vi "Get Orientation.vi"(0 "Matches (pixel)":T2(array[cluster]) {"Bounding Box"."y" format="%.2f"; "Bounding Box"."x" format="%.2f"; "Position"."y" format="%.2f"; "Position"."x" format="%.2f"; "Score" format="%.2f"; "Scale" format="%.2f"; "Angle" format="%.2f"}, 2 "Image Src":T1, 5 "error in (no error)":errorcluster, 6 "Image Dst":T1(plugin-control), 7 "y":dbl=20.0 format="%#_13g", 9 "X":dbl=100.0 format="%#_13g", 11 "yB":dbl=20.0, 13 "XB":dbl=100.0 format="%#_13g") -> (10 "Centre":dbl[][](array[numeric]) format="%.2f", 12 "Angle":sgl, 14 "Image 3":T1(plugin-control), 15 "X":sgl, 16 "no error":bool, 18 "y":sgl, 19 "错误输出":errorcluster)   [LabVIEW 2016]
uses:
  <vilib>/vision/Image Controls.llb/IMAQ Image.ctl
  <vilib>/vision/Measure.llb/Edge Options.ctl
  <vilib>/vision/Measure.llb/Edge Polarity.ctl
  <vilib>/vision/Measure.llb/Straight Edge Options.ctl
  <vilib>/vision/Measure.llb/Straight Edge Process.ctl
  <vilib>/vision/NI_Vision_Development_Module.lvlib
panel:
  out "Image 2":T1(plugin-control)
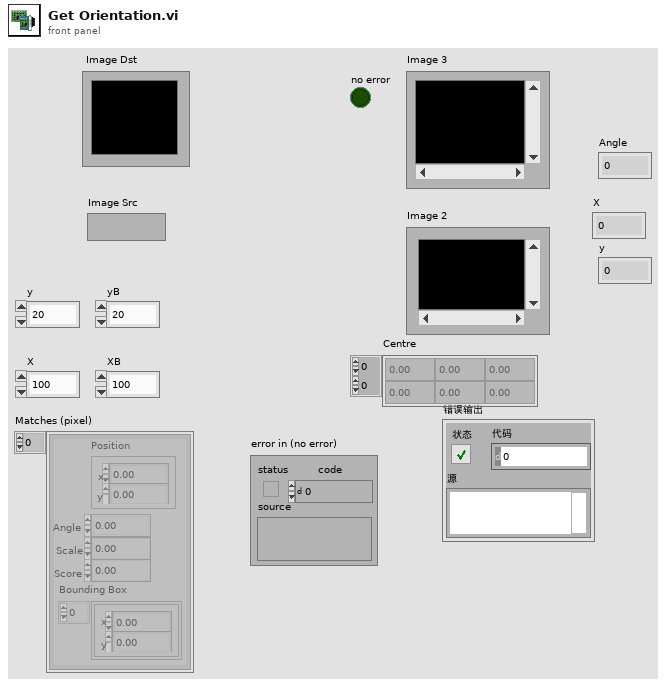
[diagram p1: front panel]
types:
  T1 = typedef "IMAQ Image.ctl" = refnum<image>
  T2 = cluster{"Position":cluster{"x":sgl, "y":sgl}, "Angle":sgl, "Scale":sgl, "Score":sgl, "Bounding Box":cluster{"x":sgl, "y":sgl}[]}[]
  T3 = cluster{"Feature":u32, "Points IDs":cluster{"GUID":string, "Index":i32}[]}[]
  T4 = typedef "IMAQ Rectangle" = cluster{"Left":i32, "Top":i32, "Right":i32, "Bottom":i32, "Rotation":dbl}
  T5 = typedef "Straight Edge Options.ctl" = cluster{"Number of Lines":i32, "Type":T6, "Min. Score":dbl, "Max. Score":dbl, "Orientation":dbl, "Angle Range":dbl, "Angle Tolerance":dbl, "Step Size":u32, "Min. SNR (db)":dbl, "Min. Points (%)":dbl, "Hough Iterations":i32}
  T6 = typedef "Straight Edge Process.ctl" = enum32{"First Edge Rake", "Best Edge Rake", "Hough Edge Rake", "First Edge Projection", "Best Edge Projection"}
  T7 = typedef "Edge Options.ctl" = cluster{"Edge Polarity":T8, "Kernel Size":u32, "Width":u32, "Minimum Edge Strength":sgl, "Interpolation Type":enum32{"Zero Order", "Bilinear", "Quadratic", "Cubic", "Bilinear Fixed"}, "Data Processing Method":enum32{"Average", "Median"}}
  T8 = typedef "Edge Polarity.ctl" = u32
  T9 = cluster{"Search Direction":u32, "Edge Options":T7, "Show Search Area":bool, "Show Search Lines":bool, "Show Edges Found":bool, "Show Result":bool, "Search Area Color":u32, "Search Lines Color":u32, "Edge Locations Color":u32, "Result Color":u32, "Overlay Group Name":string}
  T10 = typedef "Particle Parameters" = i32
  T11 = cluster{"Measurement Parameter":T10, "Range Lower Value":dbl, "Range Upper Value":dbl, "Range":bool, "Measurement Type":bool}[]
  T12 = cluster{"Position":cluster{"x":sgl, "y":sgl}, "Angle":sgl, "Scale":sgl, "Score":sgl, "Bounding Box":cluster{"x":sgl, "y":sgl}[]}
  T13 = typedef "ROI Descriptor" = cluster{"Global Rectangle":i32[], "Contours":cluster{"ID":enum32{"External", "Internal"}, "Type":u32, "Coordinates":i32[]}[]}
  T14 = cluster{"histogram":u32[], "Minimal Value":sgl, "Maximal Value":sgl, "Starting Value":sgl, "Interval Width":sgl, "Mean Value":sgl, "Standard  Variation":sgl, "Area (pixels)":i32}
  T15 = typedef "Image Type" = u32
  T16 = cluster{"Point1 (Pixels)":cluster{"X":sgl, "Y":sgl}, "Point2 (Pixels)":cluster{"X":sgl, "Y":sgl}, "Point1 (Real-World)":cluster{"X":sgl, "Y":sgl}, "Point2 (Real-World)":cluster{"X":sgl, "Y":sgl}, "Angle (Pixel)":dbl, "Angle (Real-World)":dbl, "Score":dbl, "Straightness":dbl, "Average SNR (db)":dbl, "Calibration Valid":bool}[]
  T17 = cluster{"Point1 (Pixels)":cluster{"X":sgl, "Y":sgl}, "Point2 (Pixels)":cluster{"X":sgl, "Y":sgl}, "Point1 (Real-World)":cluster{"X":sgl, "Y":sgl}, "Point2 (Real-World)":cluster{"X":sgl, "Y":sgl}, "Angle (Pixel)":dbl, "Angle (Real-World)":dbl, "Score":dbl, "Straightness":dbl, "Average SNR (db)":dbl, "Calibration Valid":bool}
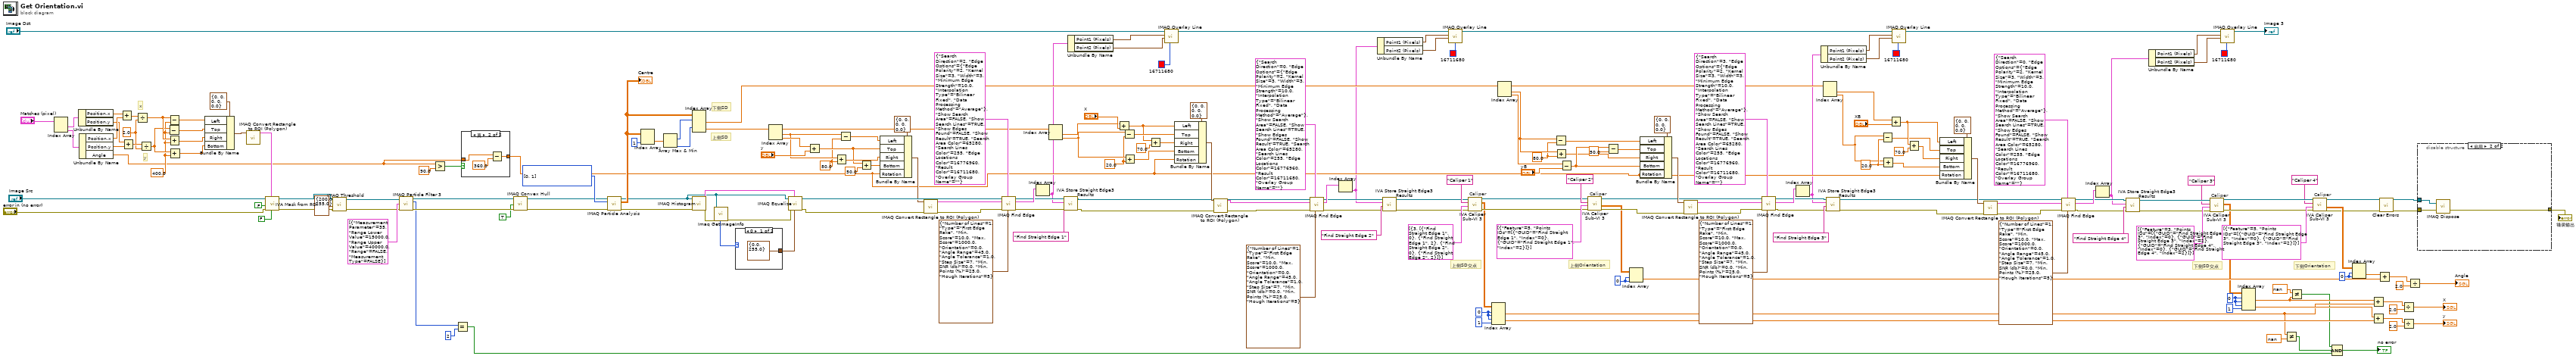
[diagram p0: block diagram]
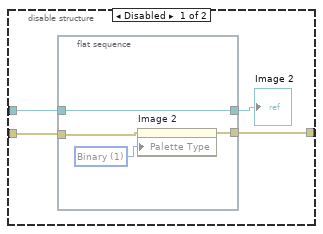
[diagram p2: hidden frame]
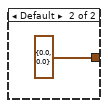
[diagram p4: hidden frame]
diagram:
  w52 = 0 ("索引 (行)")
  w50 = 0 ("索引 (行)")
  w59 = 0
  w60 = 0
  w79 = 20.0 ("y")
  w104 = 80.0 ("y")
  w106 = 20.0 ("y")
  w107 = 80.0 ("y")
  w185 = T10[] [0, 1] items=["Center of Mass X", "Center of Mass Y", "First Pixel X", "First Pixel Y", "Bounding Rect Left", "Bounding Rect Top", "Bounding Rect Right", "Bounding Rect Bottom", "Max Feret Diameter Start X", "Max Feret Diameter Start Y", "Max Feret Diameter End X", "Max Feret Diameter End Y", "Max Horiz. Segment Length Left", "Max Horiz. Segment Length Right", "Max Horiz. Segment Length Row", "-", "Bounding Rect Width", "Bounding Rect Height", "Bounding Rect Diagonal", "Perimeter", "Convex Hull Perimeter", "Holes' Perimeter", "Max Feret Diameter", "Equivalent Ellipse Major Axis", "Equivalent Ellipse Minor Axis", "Equivalent Ellipse Minor Axis (Feret)", "Equivalent Rect Long Side", "Equivalent Rect Short Side", "Equivalent Rect Diagonal", "Equivalent Rect Short Side (Feret)", "Average Horiz. Segment Length", "Average Vert. Segment Length", "Hydraulic Radius", "Waddel Disk Diameter", "-", "Area", "Holes' Area", "Particle & Holes' Area", "Convex Hull Area", "Image Area", "-", "Number of Holes", "Number of Horiz. Segments", "Number of Vert. Segments", "-", "Orientation", "Max Feret Diameter Orientation", "-", "% Area/Image Area", "% Area/(Particle & Holes' Area)", "Ratio of Equivalent Ellipse Axes", "Ratio of Equivalent Rect Sides", "-", "Elongation Factor", "Compactness Factor", "Heywood Circularity Factor", "Type Factor", "-", "Sum X", "Sum Y", "Sum XX", "Sum XY", "Sum YY", "Sum XXX", "Sum XXY", "Sum XYY", "Sum YYY", "-", "Moment of Inertia XX", "Moment of Inertia XY", "Moment of Inertia YY", "Moment of Inertia XXX", "Moment of Inertia XXY", "Moment of Inertia XYY", "Moment of Inertia YYY", "Norm. Moment of Inertia XX", "Norm. Moment of Inertia XY", "Norm. Moment of Inertia YY", "Norm. Moment of Inertia XXX", "Norm. Moment of Inertia XXY", "Norm. Moment of Inertia XYY", "Norm. Moment of Inertia YYY", "Hu Moment 1", "Hu Moment 2", "Hu Moment 3", "Hu Moment 4", "Hu Moment 5", "Hu Moment 6", "Hu Moment 7"] ("Pixel Measurements")
  w197 = sgl 400.0 ("y")
  w204 = sgl 2.0 ("y")
  # "下侧Orientation"
  # "下侧SD交点"
  # "Caliper"
  # "Caliper"
  # "上侧Orientation"
  # "上侧SD交点"
  # "Caliper"
  # "Caliper"
  # "下侧SD"
  # "上侧SD"
  # "y"
  # "x"
  n1 = Index Array(array="Matches (pixel)") -> (element #1=w212:T12, element #2=w211:T12)  [unwired: 2 in]
  n2 = Unbundle By Name(w212) -> ("Position.x"=w209:sgl, "Position.y"=w208:sgl)
  n3 = Unbundle By Name(w211) -> ("Position.x"=w210:sgl, "Position.y"=w207:sgl, "Angle"=w154:sgl)
  n4 = Add(x=w209, y=w210) -> (x+y=w206:sgl)
  n5 = Add(x=w208, y=w207) -> (x+y=w205:sgl)
  n6 = Divide(x=w206, y=w204) -> (x/y=w199:sgl)
  n7 = Divide(x=w205, y=w204) -> (x/y=w198:sgl)
  n8 = Subtract(x=w198, y=w197) -> (x-y=w200:sgl)
  n9 = Subtract(x=w199, y=w197) -> (x-y=w201:sgl)
  n10 = Add(x=w199, y=w197) -> (x+y=w196:sgl)
  n11 = Add(x=w198, y=w197) -> (x+y=w195:sgl)
  n12 = Bundle By Name(cluster=T4 {"Left"=0, "Top"=0, "Right"=0, "Bottom"=0, "Rotation"=0.0} ("Rectangle"), "Left"=w201, "Top"=w200, "Right"=w196, "Bottom"=w195) -> (w202:T4)
  n13 = call "IMAQ Convert Rectangle to ROI (Polygon)"("Rectangle"=w202) -> ("ROI Descriptor"=w194:T13)  [unwired: 7 in, 2 out]
  n14 = call <vilib>:"IVA Mask from ROI.vi"("Shrink"=FALSE ("Out / In"), "ROI Descriptor"=w194, "error in (no error)"="error in (no error)", "Out / In"=FALSE, "Image Src"="Image Src") -> ("error out"=w16:errorcluster, "Image Out"=w14:T1)  [unwired: 5 out]
  n15 = call "IMAQ Threshold"("error in (no error)"=w16, "Range"=cluster{"Lower value":sgl, "Upper value":sgl} {"Lower value"=200.0, "Upper value"=255.0}, "Image Src"=w14) -> ("error out"=w17:errorcluster, "Image Dst Out"=w15:T1)  [unwired: 7 in]
  n16 = call "IMAQ Particle Filter 3"("Image Src"=w15, "Selection Values"=T11 [{"Measurement Parameter"=35, "Range Lower Value"=15000.0, "Range Upper Value"=40000.0, "Range"=FALSE, "Measurement Type"=FALSE}], "error in (no error)"=w17) -> ("Image Dst Out"=w188:T1, "Number of Particles"=w13:i32, "error out"=w187:errorcluster)  [unwired: 10 in]
  n17 = Greater?(x=w154, y=sgl 90.0) -> (0:w155:bool)
  n18 = Equal?(x=w13, y=2) -> (x = y?=w1:bool)
  n19 = case shown="真" w155 {
    tunnel: w154 -> [w213 w214]
    tunnel: [w213 w216] -> w74
    frame False {
    }
    frame True {
      n20 = Subtract(x=w214, y=360.0 ("x")) -> (x-y=w216:dbl)
    }
  }
  n21 = call "IMAQ Convex Hull"("error in (no error)"=w187, "Connectivity 4/8 (8)"=TRUE, "Image Src"=w188) -> ("error out"=w183:errorcluster, "Image Dst Out"=w184:T1)  [unwired: 7 in]
  n22 = call "IMAQ Particle Analysis"("error in (no error)"=w183, "Pixel Measurements"=w185, "Image"=w184) -> ("error out"=w172:errorcluster, "Particle Measurements (Pixels)"=w180:dbl[][], "Image Out (duplicate)"=w171:T1)  [unwired: 3 in, 3 out]
  "Centre" <- w180
  n23 = Index Array(array=w180, index (col)=1 ("禁用的索引 (列)")) -> (element=w181:dbl[])  [unwired: 1 in]
  n24 = Array Max & Min(array=w181) -> (max index (indices)=w179:i32, min index (indices)=w178:i32)  [unwired: 2 out]
  n25 = Index Array(array=w180, index (row) #1=w179, index (row) #2=w178) -> (element #1=w82:dbl[], element #2=w144:dbl[])  [unwired: 2 in]
  n26 = call "IMAQ Histogram"("error in (no error)"=w172, "Image"=w171) -> ("error out"=w175:errorcluster, "Histogram Report"=w177:T14)  [unwired: 3 in, 5 out]
  n27 = call "Imaq GetImageInfo"("error in (no error)"=w175, "Image"=w171) -> ("error out"=w174:errorcluster, "Image Type"=w176:T15)  [unwired: 8 out]
  n28 = case "条件结构" shown="0" w176 {
    tunnel: [cluster{"Minimum":sgl, "Maximum":sgl} {"Minimum"=0.0, "Maximum"=255.0} ("Range") cluster{"Minimum":sgl, "Maximum":sgl} {"Minimum"=0.0, "Maximum"=0.0} ("Range")] -> w173
    frame 0 {
    }
    frame Default {
    }
  }
  n29 = Index Array(array=w144) -> (element #1=w161:dbl, element #2=w162:dbl)  [unwired: 2 in]
  n30 = call "IMAQ Equalize"("Range"=w173, "Histogram Report"=w177, "error in (no error)"=w174, "Image Src"=w171) -> ("error out"=w167:errorcluster, "Image Dst Out"=w170:T1)  [unwired: 2 in, 4 out]
  n31 = Add(x=w162, y="y") -> (x+y=w158:dbl)
  n32 = Add(x=w161, y=w107) -> (x+y=w160:dbl)
  n33 = Subtract(x=w161, y=w107) -> (x-y=w164:dbl)
  n34 = Add(x=w158, y=50.0) -> (x+y=w157:dbl)
  n35 = Bundle By Name(cluster=T4 {"Left"=0, "Top"=0, "Right"=0, "Bottom"=0, "Rotation"=0.0} ("Rectangle"), "Left"=w164, "Top"=w158, "Right"=w160, "Bottom"=w157, "Rotation"=w74) -> (w165:T4)
  n36 = call "IMAQ Convert Rectangle to ROI (Polygon)"("error in (no error)"=w167, "Rectangle"=w165) -> ("error out"=w152:errorcluster, "ROI Descriptor"=w153:T13)  [unwired: 6 in, 1 out]
  n37 = call "IMAQ Find Edge"("Line Fit Options"=T5 {"Number of Lines"=1, "Type"=enum."First Edge Rake", "Min. Score"=10.0, "Max. Score"=1000.0, "Orientation"=0.0, "Angle Range"=45.0, "Angle Tolerance"=1.0, "Step Size"=7, "Min. SNR (db)"=0.0, "Min. Points (%)"=25.0, "Hough Iterations"=5}, "Options"=T9 {"Search Direction"=2, "Edge Options"={"Edge Polarity"=2, "Kernel Size"=3, "Width"=3, "Minimum Edge Strength"=10.0, "Interpolation Type"=enum."Bilinear Fixed", "Data Processing Method"=enum."Average"}, "Show Search Area"=FALSE, "Show Search Lines"=TRUE, "Show Edges Found"=FALSE, "Show Result"=TRUE, "Search Area Color"=65280, "Search Lines Color"=255, "Edge Locations Color"=16776960, "Result Color"=16711680, "Overlay Group Name"=""}, "error in (no error)"=w152, "ROI Descriptor"=w153, "Image"=w170) -> ("error out"=w148:errorcluster, "Straight Edges"=w151:T16, "Image Out"=w150:T1)  [unwired: 1 in, 3 out]
  n38 = Index Array(array=w151) -> (element=w40:T17)  [unwired: 1 in]
  n39 = Index Array(array=w144) -> (element #1=w140:dbl, element #2=w143:dbl)  [unwired: 2 in]
  n40 = call <vilib>:"IVA Store Straight Edge3 Results.vi"("error in (no error)"=w148, "Step Name"="Find Straight Edge 1", "Straight Edge"=w40, "Image in"=w150) -> ("error out"=w147:errorcluster, "Image dup"=w135:T1)  [unwired: 1 in, 5 out]
  n41 = Unbundle By Name(w40) -> ("Point1 (Pixels)"=w39:cluster{"X":sgl, "Y":sgl}, "Point2 (Pixels)"=w38:cluster{"X":sgl, "Y":sgl})
  n42 = Add(x=w140, y="X") -> (x+y=w123:dbl)
  n43 = Subtract(x=w143, y=w106) -> (x-y=w124:dbl)
  n44 = Add(x=w143, y=w106) -> (x+y=w138:dbl)
  n45 = Add(x=w123, y=70.0) -> (x+y=w139:dbl)
  n46 = call "IMAQ Overlay Line"("Color"=u32 16711680, "End Point"=w38, "Start Point"=w39, "Image"="Image Dst") -> ("Image Out"=w32:T1)  [unwired: 6 in, 1 out]
  n47 = Bundle By Name(cluster=T4 {"Left"=0, "Top"=0, "Right"=0, "Bottom"=0, "Rotation"=0.0} ("Rectangle"), "Left"=w123, "Top"=w124, "Right"=w139, "Bottom"=w138, "Rotation"=w74) -> (w145:T4)
  n48 = call "IMAQ Convert Rectangle to ROI (Polygon)"("error in (no error)"=w147, "Rectangle"=w145) -> ("error out"=w136:errorcluster, "ROI Descriptor"=w137:T13)  [unwired: 6 in, 1 out]
  n49 = call "IMAQ Find Edge"("Line Fit Options"=T5 {"Number of Lines"=1, "Type"=enum."First Edge Rake", "Min. Score"=10.0, "Max. Score"=1000.0, "Orientation"=0.0, "Angle Range"=45.0, "Angle Tolerance"=1.0, "Step Size"=7, "Min. SNR (db)"=0.0, "Min. Points (%)"=25.0, "Hough Iterations"=5}, "Options"=T9 {"Search Direction"=0, "Edge Options"={"Edge Polarity"=2, "Kernel Size"=3, "Width"=3, "Minimum Edge Strength"=10.0, "Interpolation Type"=enum."Bilinear Fixed", "Data Processing Method"=enum."Average"}, "Show Search Area"=FALSE, "Show Search Lines"=TRUE, "Show Edges Found"=FALSE, "Show Result"=TRUE, "Search Area Color"=65280, "Search Lines Color"=255, "Edge Locations Color"=16776960, "Result Color"=16711680, "Overlay Group Name"=""}, "error in (no error)"=w136, "ROI Descriptor"=w137, "Image"=w135) -> ("error out"=w126:errorcluster, "Straight Edges"=w132:T16, "Image Out"=w131:T1)  [unwired: 1 in, 3 out]
  n50 = Index Array(array=w132) -> (element=w35:T17)  [unwired: 1 in]
  n51 = Unbundle By Name(w35) -> ("Point1 (Pixels)"=w34:cluster{"X":sgl, "Y":sgl}, "Point2 (Pixels)"=w33:cluster{"X":sgl, "Y":sgl})
  n52 = call <vilib>:"IVA Store Straight Edge3 Results.vi"("error in (no error)"=w126, "Step Name"="Find Straight Edge 2", "Straight Edge"=w35, "Image in"=w131) -> ("error out"=w125:errorcluster, "Image dup"=w127:T1)  [unwired: 1 in, 5 out]
  n53 = call "IMAQ Overlay Line"("Color"=u32 16711680, "End Point"=w33, "Start Point"=w34, "Image"=w32) -> ("Image Out"=w27:T1)  [unwired: 6 in, 1 out]
  n54 = call <vilib>:"IVA Caliper Sub-VI 3.vi"("error in"=w125, "Parameters"=T3 [{"Feature"=3, "Points IDs"=[{"GUID"="Find Straight Edge 1", "Index"=0}, {"GUID"="Find Straight Edge 1", "Index"=2}, {"GUID"="Find Straight Edge 2", "Index"=0}, {"GUID"="Find Straight Edge 2", "Index"=2}]}], "Step Name"="Caliper 1", "Image In"=w127) -> ("error out"=w119:errorcluster, "Results (Pixels)"=w53:sgl[][], "Image Out"=w118:T1)  [unwired: 1 in, 4 out]
  n55 = Index Array(array=w53, index (row) #1=w52, index (col) #1=w52, index (row) #2=w52, index (col) #2=1 ("索引 (行)")) -> (element #1=w5:sgl, element #2=w43:sgl)
  n56 = Index Array(array=w82) -> (element #1=w105:dbl, element #2=w101:dbl)  [unwired: 2 in]
  n57 = Subtract(x=w105, y=w104) -> (x-y=w97:dbl)
  n58 = Add(x=w105, y=w104) -> (x+y=w96:dbl)
  n59 = Subtract(x=w101, y="yB") -> (x-y=w99:dbl)
  n60 = call <vilib>:"IVA Caliper Sub-VI 3.vi"("error in"=w119, "Parameters"=T3 [{"Feature"=5, "Points IDs"=[{"GUID"="Find Straight Edge 1", "Index"=0}, {"GUID"="Find Straight Edge 1", "Index"=2}]}], "Step Name"="Caliper 2", "Image In"=w118) -> ("error out"=w102:errorcluster, "Results (Calibrated)"=w61:sgl[][], "Image Out"=w103:T1)  [unwired: 1 in, 4 out]
  n61 = Subtract(x=w99, y=50.0) -> (x-y=w98:dbl)
  n62 = Index Array(array=w61, index (row)=w60, index (col)=w60) -> (element=w57:sgl)
  n63 = Bundle By Name(cluster=T4 {"Left"=0, "Top"=0, "Right"=0, "Bottom"=0, "Rotation"=0.0} ("Rectangle"), "Left"=w97, "Top"=w98, "Right"=w96, "Bottom"=w99, "Rotation"=w74) -> (w114:T4)
  n64 = call "IMAQ Convert Rectangle to ROI (Polygon)"("error in (no error)"=w102, "Rectangle"=w114) -> ("error out"=w112:errorcluster, "ROI Descriptor"=w113:T13)  [unwired: 6 in, 1 out]
  n65 = call "IMAQ Find Edge"("Line Fit Options"=T5 {"Number of Lines"=1, "Type"=enum."First Edge Rake", "Min. Score"=10.0, "Max. Score"=1000.0, "Orientation"=0.0, "Angle Range"=45.0, "Angle Tolerance"=1.0, "Step Size"=7, "Min. SNR (db)"=0.0, "Min. Points (%)"=25.0, "Hough Iterations"=5}, "Options"=T9 {"Search Direction"=3, "Edge Options"={"Edge Polarity"=2, "Kernel Size"=3, "Width"=3, "Minimum Edge Strength"=10.0, "Interpolation Type"=enum."Bilinear Fixed", "Data Processing Method"=enum."Average"}, "Show Search Area"=FALSE, "Show Search Lines"=TRUE, "Show Edges Found"=FALSE, "Show Result"=TRUE, "Search Area Color"=65280, "Search Lines Color"=255, "Edge Locations Color"=16776960, "Result Color"=16711680, "Overlay Group Name"=""}, "error in (no error)"=w112, "ROI Descriptor"=w113, "Image"=w103) -> ("error out"=w108:errorcluster, "Straight Edges"=w111:T16, "Image Out"=w110:T1)  [unwired: 1 in, 3 out]
  n66 = Index Array(array=w111) -> (element=w26:T17)  [unwired: 1 in]
  n67 = Unbundle By Name(w26) -> ("Point1 (Pixels)"=w28:cluster{"X":sgl, "Y":sgl}, "Point2 (Pixels)"=w29:cluster{"X":sgl, "Y":sgl})
  n68 = Index Array(array=w82) -> (element #1=w73:dbl, element #2=w72:dbl)  [unwired: 2 in]
  n69 = call <vilib>:"IVA Store Straight Edge3 Results.vi"("error in (no error)"=w108, "Step Name"="Find Straight Edge 3", "Straight Edge"=w26, "Image in"=w110) -> ("error out"=w83:errorcluster, "Image dup"=w84:T1)  [unwired: 1 in, 5 out]
  n70 = Subtract(x=w72, y=w79) -> (x-y=w77:dbl)
  n71 = Add(x=w72, y=w79) -> (x+y=w75:dbl)
  n72 = Add(x=w73, y="XB") -> (x+y=w78:dbl)
  n73 = call "IMAQ Overlay Line"("Color"=u32 16711680, "End Point"=w29, "Start Point"=w28, "Image"=w27) -> ("Image Out"=w21:T1)  [unwired: 6 in, 1 out]
  n74 = Add(x=w78, y=70.0) -> (x+y=w76:dbl)
  n75 = Bundle By Name(cluster=T4 {"Left"=0, "Top"=0, "Right"=0, "Bottom"=0, "Rotation"=0.0} ("Rectangle"), "Left"=w78, "Top"=w77, "Right"=w76, "Bottom"=w75, "Rotation"=w74) -> (w91:T4)
  n76 = call "IMAQ Convert Rectangle to ROI (Polygon)"("error in (no error)"=w83, "Rectangle"=w91) -> ("error out"=w89:errorcluster, "ROI Descriptor"=w90:T13)  [unwired: 6 in, 1 out]
  n77 = call "IMAQ Find Edge"("Line Fit Options"=T5 {"Number of Lines"=1, "Type"=enum."First Edge Rake", "Min. Score"=10.0, "Max. Score"=1000.0, "Orientation"=0.0, "Angle Range"=45.0, "Angle Tolerance"=1.0, "Step Size"=7, "Min. SNR (db)"=0.0, "Min. Points (%)"=25.0, "Hough Iterations"=5}, "Options"=T9 {"Search Direction"=0, "Edge Options"={"Edge Polarity"=2, "Kernel Size"=3, "Width"=3, "Minimum Edge Strength"=10.0, "Interpolation Type"=enum."Bilinear Fixed", "Data Processing Method"=enum."Average"}, "Show Search Area"=FALSE, "Show Search Lines"=TRUE, "Show Edges Found"=FALSE, "Show Result"=TRUE, "Search Area Color"=65280, "Search Lines Color"=255, "Edge Locations Color"=16776960, "Result Color"=16711680, "Overlay Group Name"=""}, "error in (no error)"=w89, "ROI Descriptor"=w90, "Image"=w84) -> ("error out"=w85:errorcluster, "Straight Edges"=w88:T16, "Image Out"=w87:T1)  [unwired: 1 in, 3 out]
  n78 = Index Array(array=w88) -> (element=w23:T17)  [unwired: 1 in]
  n79 = call <vilib>:"IVA Store Straight Edge3 Results.vi"("error in (no error)"=w85, "Step Name"="Find Straight Edge 4", "Straight Edge"=w23, "Image in"=w87) -> ("error out"=w66:errorcluster, "Image dup"=w67:T1)  [unwired: 1 in, 5 out]
  n80 = Unbundle By Name(w23) -> ("Point1 (Pixels)"=w22:cluster{"X":sgl, "Y":sgl}, "Point2 (Pixels)"=w25:cluster{"X":sgl, "Y":sgl})
  n81 = call <vilib>:"IVA Caliper Sub-VI 3.vi"("error in"=w66, "Parameters"=T3 [{"Feature"=3, "Points IDs"=[{"GUID"="Find Straight Edge 3", "Index"=0}, {"GUID"="Find Straight Edge 3", "Index"=2}, {"GUID"="Find Straight Edge 4", "Index"=0}, {"GUID"="Find Straight Edge 4", "Index"=2}]}], "Step Name"="Caliper 3", "Image In"=w67) -> ("error out"=w69:errorcluster, "Results (Pixels)"=w54:sgl[][], "Image Out"=w68:T1)  [unwired: 1 in, 4 out]
  n82 = call "IMAQ Overlay Line"("Color"=u32 16711680, "End Point"=w25, "Start Point"=w22, "Image"=w21) -> ("Image Out"=→"Image 3":T1)  [unwired: 6 in, 1 out]
  n83 = Index Array(array=w54, index (row) #1=w50, index (col) #1=w50, index (row) #2=w50, index (col) #2=1 ("索引 (行)")) -> (element #1=w7:sgl, element #2=w44:sgl)
  n84 = Not Equal?(x=w5, y=sgl nan ("output string")) -> (x != y?=w3:bool)
  n85 = Not Equal?(x=sgl nan ("output string"), y=w7) -> (x != y?=w4:bool)
  n86 = call <vilib>:"IVA Caliper Sub-VI 3.vi"("error in"=w69, "Parameters"=T3 [{"Feature"=5, "Points IDs"=[{"GUID"="Find Straight Edge 3", "Index"=0}, {"GUID"="Find Straight Edge 3", "Index"=2}]}], "Step Name"="Caliper 4", "Image In"=w68) -> ("error out"=w10:errorcluster, "Results (Calibrated)"=w62:sgl[][], "Image Out"=w63:T1)  [unwired: 1 in, 4 out]
  n87 = Compound Arithmetic op=AND ("复合运算")(w4, w3, w1) -> (→"no error":bool)
  n88 = Index Array(array=w62, index (row)=w59, index (col)=w59) -> (element=w58:sgl)
  n89 = Add(x=w7, y=w5) -> (x+y=w47:sgl)
  n90 = Add(x=w44, y=w43) -> (x+y=w46:sgl)
  n91 = Add(x=w58, y=w57) -> (x+y=w56:sgl)
  n92 = call <vilib>:"Clear Errors.vi"("error in (no error)"=w10) -> ("error out"=w9:errorcluster)  [unwired: 5 in, 1 out]
  n93 = Divide(x=w47, y=sgl 2.0) -> (x/y=→"X":sgl)
  n94 = Divide(x=w46, y=sgl 2.0) -> (x/y=→"y":sgl)
  n95 = Divide(x=w56, y=sgl 2.0) -> (x/y=→"Angle":sgl)
  n96 = disable-structure shown="启用" {
    disable-tunnel: [w222 w227] -> w122
    disable-tunnel: w63 -> [w220 w229]
    disable-tunnel: w9 -> [w219 w228]
    frame Disabled {
      n97 = flat-sequence {
        tunnel: [w225] -> w222
        tunnel: w219 -> [w224]
        tunnel: w220 -> [w223]
        tunnel: [w223] -> w221
        frame #0 {
          w226 = u32 1 items=["Grayscale", "Binary", "Gradient", "Rainbow", "Temperature", "User Defined", "Binary 16 Bit", "Gradient 16 Bit", "Rainbow 16 Bit", "Temperature 16 Bit", "User Defined 16 Bit"] ("Palette:Palette Type")
          n98 = property on="Image 2" class="ImageControl"(error in=w224, "Palette Type"=w226) -> (error out=w225:errorcluster)  [unwired: 1 in, 1 out]
        }
      }
      "Image 2" <- w221
    }
    frame Enabled {
      n99 = call "IMAQ Dispose"("Image"=w229, "error in (no error)"=w228) -> ("error out"=w227:errorcluster)  [unwired: 4 in]
    }
  }
  "错误输出" <- w122
